vi "Analyze GB - Detail (2).vi"(8 "Integer Tolerance":dbl=0.1, 10 "Find Integer Rep?":bool, 11 "Grain Boundary Definition":T1={"Grain 1 Orientation"=[1.0, 1.0, 1.0], "Grain 2 Orientation"=[1.0, 1.0, 1.0], "Twist Angle (Deg)"=60.0, "Translation Vector"=[0.0, 0.0, 0.0]}) -> (0 "STEM Viewing Angles":dbl[][](array[numeric]), 1 "Misorientation":T3={"Misorientation Angle"=0.0, "Misorientation Axis, o"=[1.0, 1.0, 1.0], "Misorientation Matrix"=[]}, 2 "Grain 2 Integers":dbl[](array[numeric])=[1.0, 1.0, 1.0], 3 "Grain 1 Integers":dbl[](array[numeric])=[1.0, 1.0, 1.0], 4 "Tilt Angle (Deg)":dbl, 5 "Suggested view direction":dbl[](array[numeric])=[1.0, 1.0, 1.0], 6 "GB Name":string, 7 "STEM Viewable?":bool)   [LabVIEW 2010]
uses:
  <vilib>/Analysis/NI_AALPro.lvlib
  <vilib>/Analysis/NI_AALBase.lvlib
  <vilib>/Analysis/_algsub.llb/Real Matrix Trace.vi
  <vilib>/Analysis/baseanly.llb/Real A x B.vi
  <vilib>/Analysis/Matrix/Datatypes/RealMatrix.ctl
  <vilib>/Analysis/Matrix/NI_Matrix.lvlib
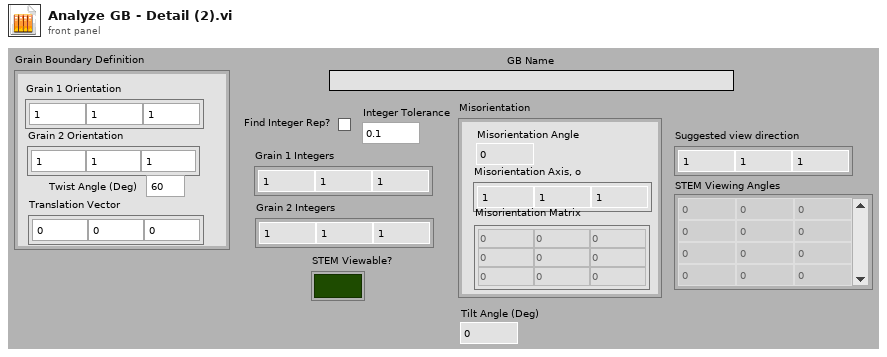
[diagram p1: front panel]
types:
  T1 = cluster{"Grain 1 Orientation":dbl[], "Grain 2 Orientation":dbl[], "Twist Angle (Deg)":dbl, "Translation Vector":dbl[]}
  T2 = typedef "NI_Matrix.lvlib/RealMatrix.ctl" = dbl[][]
  T3 = cluster{"Misorientation Angle":dbl, "Misorientation Axis, o":dbl[], "Misorientation Matrix":T2}
  T4 = cluster{"Grain 1 Orientation":dbl[], "Grain 2 Orientation":dbl[], "Twist Angle (Deg)":dbl}
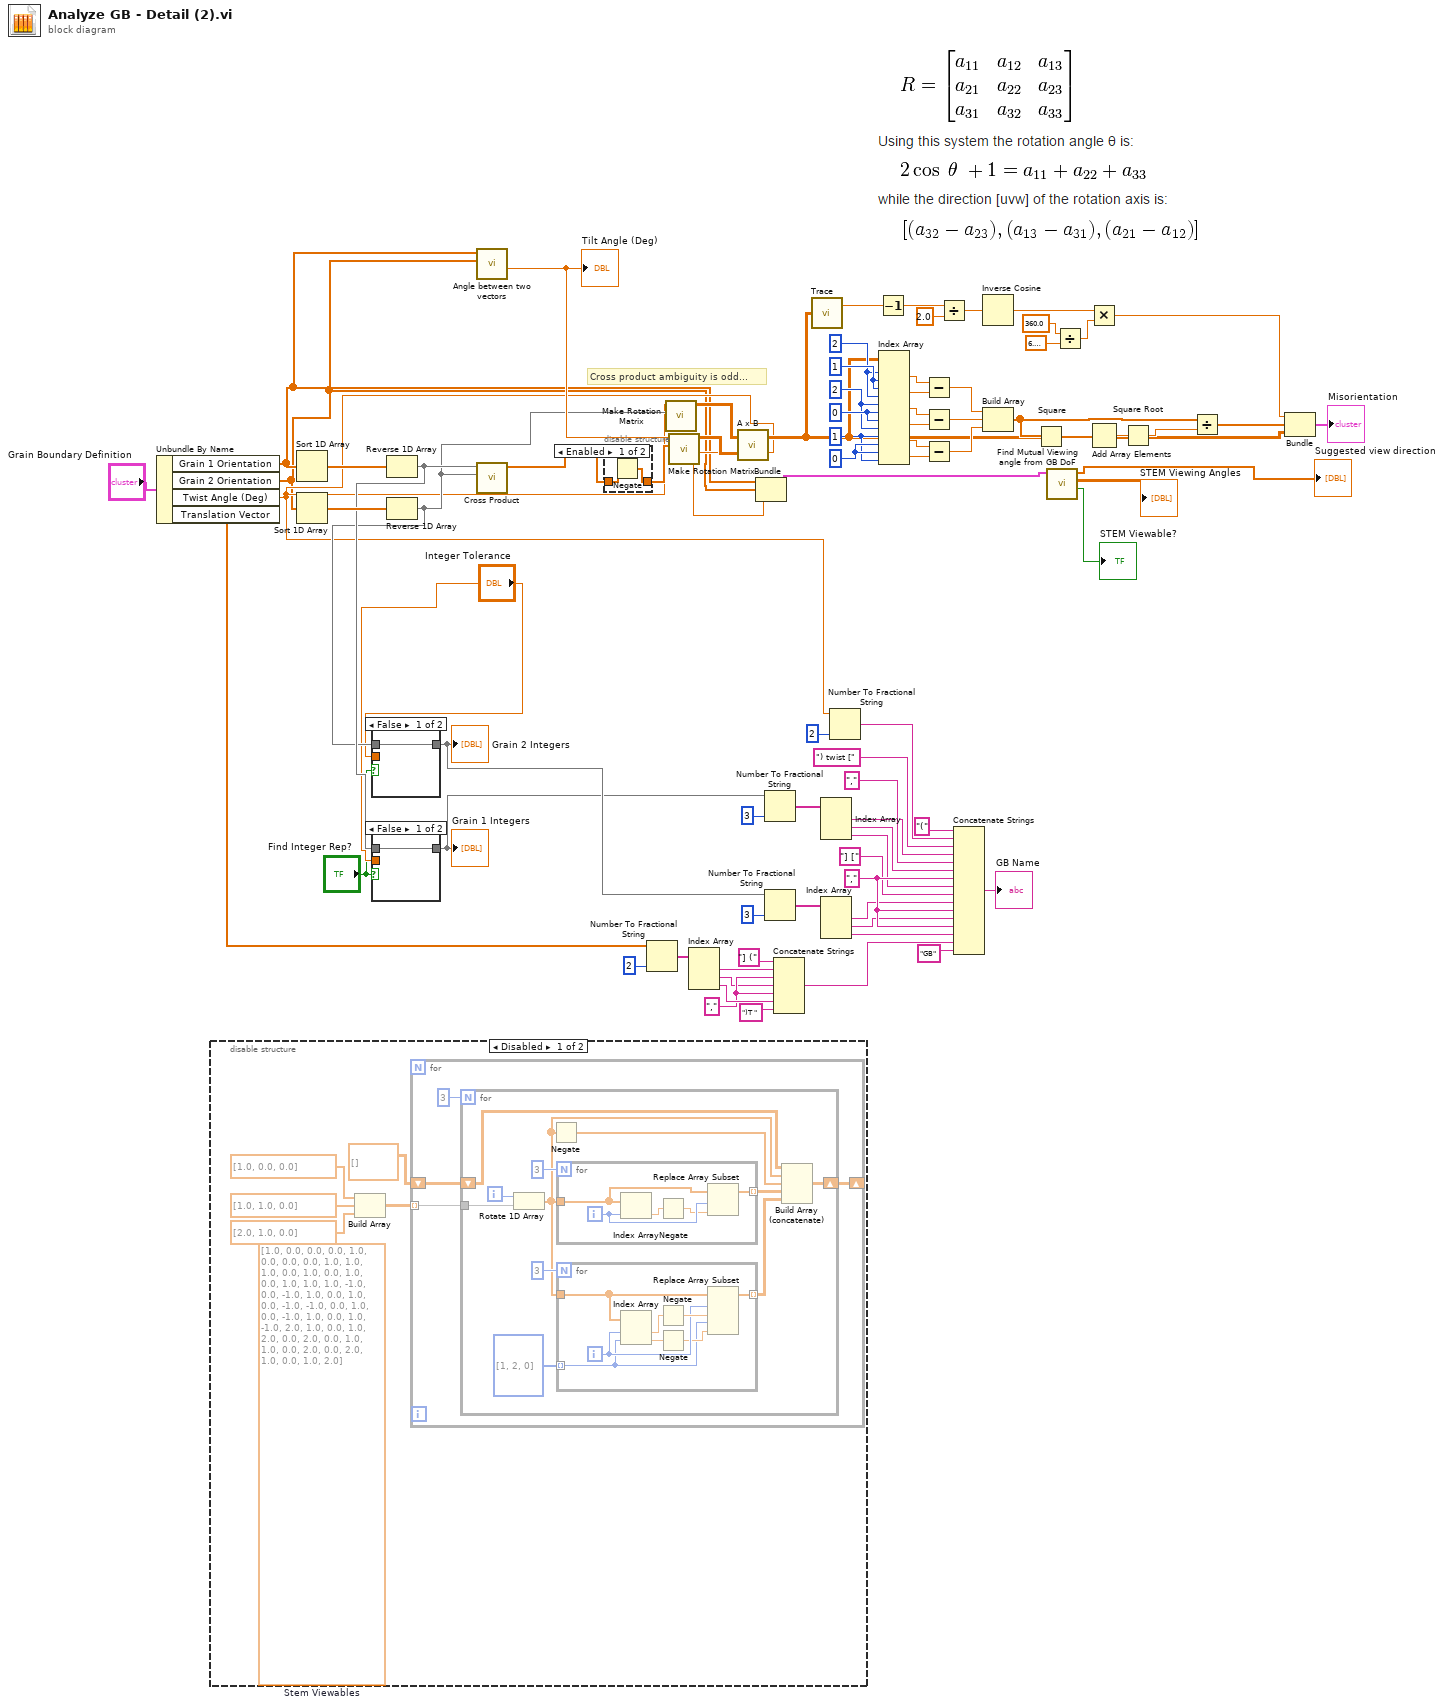
[diagram p0: block diagram]
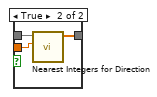
[diagram p3: hidden frame]
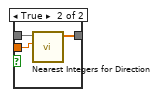
[diagram p4: hidden frame]
diagram:
  w37 = "," ("string")
  w30 = "," ("string")
  w62 = 0 ("index (row)")
  w61 = 1 ("index (row)")
  w64 = 0 ("disabled index (col)")
  w63 = 2 ("index (row)")
  w66 = 1 ("disabled index (col)")
  w65 = 2 ("index (row)")
  # "Cross product ambiguity is odd..."
  n1 = Unbundle By Name("Grain Boundary Definition") -> ("Grain 1 Orientation"=w2:dbl[], "Grain 2 Orientation"=w1:dbl[], "Twist Angle (Deg)"=w7:dbl, "Translation Vector"=w8:dbl[])
  n2 = disable-structure shown="Disabled" {
    frame Disabled {
      (unwired) dbl[][] [[1.0, 0.0, 0.0], [0.0, 1.0, 0.0], [0.0, 0.0, 1.0], [1.0, 1.0, 0.0], [1.0, 0.0, 1.0], [0.0, 1.0, 1.0], [1.0, -1.0, 0.0], [-1.0, 1.0, 0.0], [1.0, 0.0, -1.0], [-1.0, 0.0, 1.0], [0.0, -1.0, 1.0], [0.0, 1.0, -1.0], [2.0, 1.0, 0.0], [1.0, 2.0, 0.0], [2.0, 0.0, 1.0], [1.0, 0.0, 2.0], [0.0, 2.0, 1.0], [0.0, 1.0, 2.0]]  # Stem Viewables
      n3 = Build Array(dbl[] [1.0, 0.0, 0.0] ("Grain 1 Orientation 2"), dbl[] [1.0, 1.0, 0.0] ("Grain 1 Orientation 2"), dbl[] [2.0, 1.0, 0.0] ("Grain 1 Orientation 2")) -> (w83:dbl[][])
      n4 = for {
        tunnel: w83 -> [w89] mode=indexing
        shift-right: [w88] -> _
        shift-left: dbl[][] [] -> [w87]
        n5 = for {
          N: 3 -> [_]
          tunnel: w89 -> [w101]
          shift-right: [w95] -> w88
          shift-left: w87 -> [w94]
          i -> [w100]
          n6 = Rotate 1D Array(1:w101, 2:w100) -> (0:w91:dbl[])
          n7 = Negate(x=w91) -> (-x=w92:dbl[])
          n8 = for {
            N: 3 -> [_]
            tunnel: w91 -> [w113]
            tunnel: [w110] -> w97 mode=indexing
            i -> [w112]
            n9 = Index Array(array=w113, index=w112) -> (element=w114:dbl)
            n10 = Negate(x=w114) -> (-x=w111:dbl)
            n11 = Replace Array Subset(array=w113, new element=w111, index=w112) -> (w110:dbl[])
          }
          n12 = for {
            N: 3 -> [_]
            tunnel: w91 -> [w108]
            tunnel: [w105] -> w96 mode=indexing
            tunnel: i32[] [1, 2, 0] -> [w102] mode=indexing
            i -> [w104]
            n13 = Index Array(array=w108, index #1=w104, index #2=w102) -> (element #1=w109:dbl, element #2=w106:dbl)
            n14 = Negate(x=w109) -> (-x=w107:dbl)
            n15 = Negate(x=w106) -> (-x=w103:dbl)
            n16 = Replace Array Subset(array=w108, new element #1=w107, index #1=w104, new element #2=w103, index #2=w102) -> (w105:dbl[])
          }
          n17 = Build Array (concatenate)(w94, w91, w92, w97, w96) -> (w95:dbl[][])
        }
      }
    }
    frame Enabled {
    }
  }
  n18 = Sort 1D Array(array=w2) -> (sorted array=w81:dbl[])
  n19 = Sort 1D Array(array=w1) -> (sorted array=w80:dbl[])
  n20 = Reverse 1D Array(array=w81) -> (reversed array=w55:dbl[])
  n21 = case shown="False" "Find Integer Rep?" {
    tunnel: [w115 w118] -> w9
    tunnel: w55 -> [w115 w117]
    tunnel: "Integer Tolerance" -> [_ w116]
    frame False {
    }
    frame True {
      n22 = call "Nearest Integers for Direction.vi"("Tolerance"=w116, "Direction"=w117) -> ("Nearest Integer Directions"=w118:dbl[])  [unwired: 8 in, 1 out]
    }
  }
  "Grain 1 Integers" <- w9
  n23 = Reverse 1D Array(array=w80) -> (reversed array=w50:dbl[])
  n24 = case shown="False" "Find Integer Rep?" {
    tunnel: [w119 w122] -> w10
    tunnel: w50 -> [w119 w121]
    tunnel: "Integer Tolerance" -> [_ w120]
    frame False {
    }
    frame True {
      n25 = call "Nearest Integers for Direction.vi"("Tolerance"=w120, "Direction"=w121) -> ("Nearest Integer Directions"=w122:dbl[])  [unwired: 8 in, 1 out]
    }
  }
  "Grain 2 Integers" <- w10
  n26 = call "Angle between two vectors.vi"("Vector 2"=w1, "Vector 1"=w2) -> ("Angle (Degrees)"=w71:dbl)  [unwired: 7 in, 2 out]
  "Tilt Angle (Deg)" <- w71
  n27 = call <vilib>:"Cross Product.vi"("B Vector"=w50, "A Vector"=w55) -> ("Cross Product"=w42:dbl[])  [unwired: 8 in, 1 out]
  n28 = disable-structure shown="Enabled" {
    disable-tunnel: w42 -> [w124 w125]
    disable-tunnel: [w123 w125] -> w41
    frame Enabled {
      n29 = Negate(x=w124) -> (-x=w123:dbl[])
    }
    frame Disabled {
    }
  }
  n30 = Number To Fractional String(number=w8, precision (6)=i16 2) -> (F-format string=w33:string[])  [unwired: 2 in]
  n31 = call "Make Rotation Matrix.vi"("Rotation Axis"=w50, "Rotation Angle (Degree)"=w7) -> ("Rotation Matrix"=w43:T2)  [unwired: 9 in]
  n32 = call "Make Rotation Matrix.vi"("Rotation Axis"=w41, "Rotation Angle (Degree)"=w71) -> ("Rotation Matrix"=w44:T2)  [unwired: 9 in]
  n33 = Index Array(array=w33) -> (element #1=w34:string, element #2=w36:string, element #3=w38:string)  [unwired: 3 in]
  n34 = call-poly <vilib>:"A x B.vi"("B"=w44, "A"=w43) -> ("A x B"=w46:T2)  [unwired: 1 out]
  n35 = Bundle("Grain 1 Orientation"=w2, "Grain 2 Orientation"=w1, "Twist Angle (Deg)"=w7) -> (w6:T4)  [unwired: 1 in]
  n36 = Number To Fractional String(number=w9, precision (6)=i16 3) -> (F-format string=w17:string[])  [unwired: 2 in]
  n37 = Number To Fractional String(number=w10, precision (6)=i16 3) -> (F-format string=w15:string[])  [unwired: 2 in]
  n38 = Concatenate Strings("] (" ("string"), w34, w37, w36, w37, w38, ")T " ("string")) -> (w14:string)
  n39 = call-poly <vilib>:"Trace.vi"("Input Matrix"=w46) -> ("trace"=w79:dbl)  [unwired: 1 out]
  n40 = Index Array(array=w17) -> (element #1=w23:string, element #2=w25:string, element #3=w26:string)  [unwired: 3 in]
  n41 = Index Array(array=w15) -> (element #1=w28:string, element #2=w29:string, element #3=w31:string)  [unwired: 3 in]
  n42 = Number To Fractional String(number=w7, precision (6)=i16 2) -> (F-format string=w21:string)  [unwired: 2 in]
  n43 = Decrement(x=w79) -> (x-1=w78:dbl)
  n44 = Index Array(array=w46, index (row) #1=w65, index (col) #1=w66, index (row) #2=w66, index (col) #2=w65, index (row) #3=w63, index (col) #3=w64, index (row) #4=w64, index (col) #4=w63, index (row) #5=w61, index (col) #5=w62, index (row) #6=w62, index (col) #6=w61) -> (element #1=w70:dbl, element #2=w69:dbl, element #3=w68:dbl, element #4=w67:dbl, element #5=w60:dbl, element #6=w59:dbl)
  n45 = Subtract(x=w70, y=w69) -> (x-y=w58:dbl)
  n46 = Subtract(x=w68, y=w67) -> (x-y=w57:dbl)
  n47 = Subtract(x=w60, y=w59) -> (x-y=w56:dbl)
  n48 = Divide(x=w78, y=2.0) -> (x/y=w76:dbl)
  n49 = Concatenate Strings("(" ("string"), w21, ") twist [" ("string"), w23, "," ("string"), w25, w30, w26, "] [" ("string"), w28, w30, w29, w30, w31, w14, "GB" ("string")) -> (→"GB Name":string)
  n50 = Inverse Cosine(1:w76) -> (0:w72:dbl)
  n51 = Build Array(w58, w57, w56) -> (w51:dbl[])
  n52 = Square(x=w51) -> (x^2=w52:dbl[])
  n53 = call "Find Mutual Viewing angle from GB DoF.vi"("Grain Boundary Macro DoF"=w6) -> ("STEM Viewable?"=→"STEM Viewable?":bool, "STEM Viewing Angles"=→"STEM Viewing Angles":dbl[][], "Mutual Viewing Angle"=→"Suggested view direction":dbl[])  [unwired: 8 in]
  n54 = Divide(x=360.0, y=6.283185307179586) -> (x/y=w75:dbl)
  n55 = Multiply(x=w72, y=w75) -> (x*y=w48:dbl)
  n56 = Add Array Elements(numeric array=w52) -> (sum=w53:dbl)
  n57 = Square Root(x=w53) -> (sqrt(x)=w54:dbl)
  n58 = Divide(x=w51, y=w54) -> (x/y=w47:dbl[])
  n59 = Bundle(w48, w47, "A x B"=w46) -> (→"Misorientation":cluster{dbl, dbl[], "A x B":T2})  [unwired: 1 in]
